vi "VT100Codes.vi"(10 "read buffer":string="\u001b[0m\u001b[01;34mmicropython-serial-0.3\u001b[0m         \u001b[01;34mrequests-2.22.0\u001b[0m\n\u001b[01;31mmicropython-serial-0.3.tar.gz\u001b[0m  \u001b[01;31mrequests-2.22.0.tar.gz\u001b[0m\nrobot@ev3dev:~$ ", 11 "Console In":string="\r\n\r\nLinux ev3dev 4.14.117-ev3dev-2.3.4-ev3 #1 PREEMPT Thu May 9 15:13:01 CDT 2019 armv5tejl\r\n             _____     _\r\n   _____   _|___ /  __| | _____   __\r\n  / _ \\ \\ / / |_ \\ / _` |/ _ \\ \\ / /\r\n |  __/\\ V / ___) | (_| |  __/\\ V /\r\n  \\___| \\_/ |____/ \\__,_|\\___| \\_/\r\n\r\nDebian stretch on LEGO MINDSTORMS EV3!\r\nLast login: Thu Feb 13 18:25:48 2020 from 130.64.189.217\r\r\nrobot@ev3dev:~$ \r\nrobot@ev3dev:~$ \r\nrobot@ev3dev:~$ brickrun -r --  pybricks-micropython\r\nPybricks MicroPython fc828f94 on 2020-01-30; linux version\r\nUse Ctrl-D to exit, Ctrl-E for paste mode\r\n>>> \nrobot@ev3dev:~$ ls\n") -> (3 "Console Out":string="\r\n\r\nLinux ev3dev 4.14.117-ev3dev-2.3.4-ev3 #1 PREEMPT Thu May 9 15:13:01 CDT 2019 armv5tejl\r\n             _____     _\r\n   _____   _|___ /  __| | _____   __\r\n  / _ \\ \\ / / |_ \\ / _` |/ _ \\ \\ / /\r\n |  __/\\ V / ___) | (_| |  __/\\ V /\r\n  \\___| \\_/ |____/ \\__,_|\\___| \\_/\r\n\r\nDebian stretch on LEGO MINDSTORMS EV3!\r\nLast login: Thu Feb 13 18:25:48 2020 from 130.64.189.217\r\r\nrobot@ev3dev:~$ \r\nrobot@ev3dev:~$ \r\nrobot@ev3dev:~$ brickrun -r --  pybricks-micropython\r\nPybricks MicroPython fc828f94 on 2020-01-30; linux version\r\nUse Ctrl-D to exit, Ctrl-E for paste mode\r\n>>> ")   [LabVIEW 2020]
uses:
  ColorText/ColorGlobals.vi
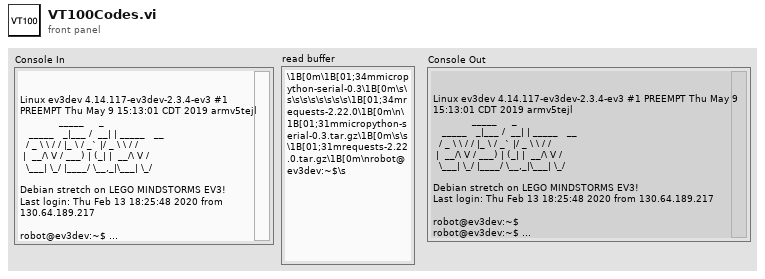
[diagram p1: front panel]
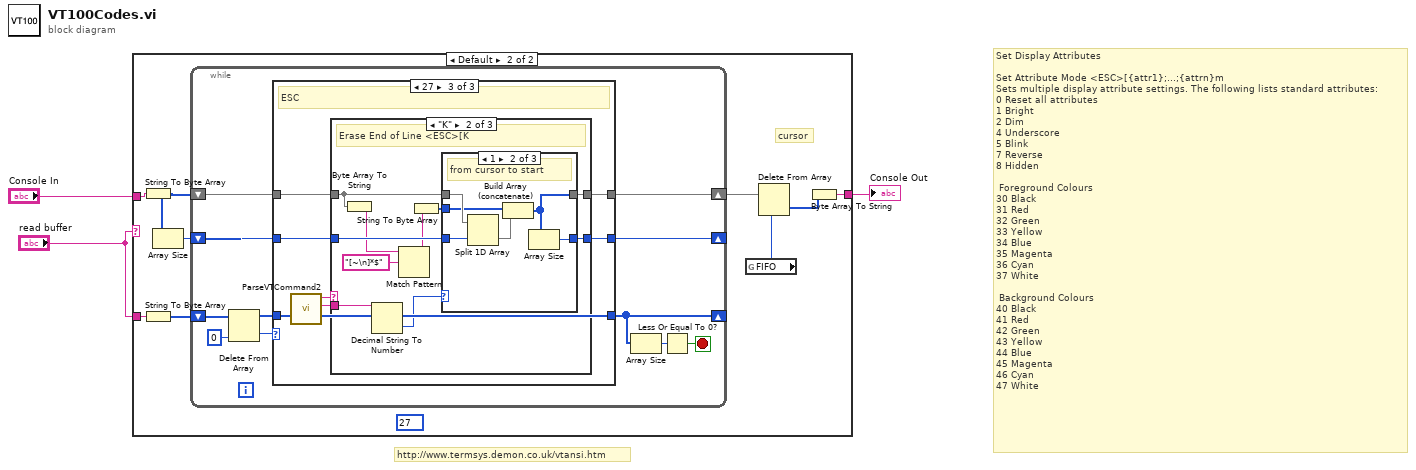
[diagram p0: block diagram]
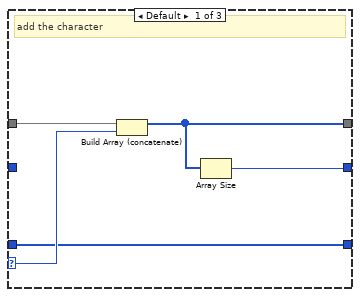
[diagram p3: hidden frame]
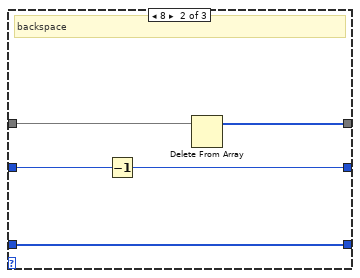
[diagram p4: hidden frame]
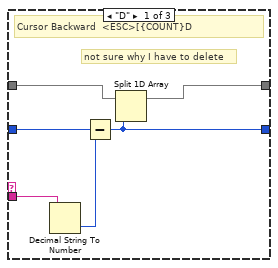
[diagram p5: hidden frame]
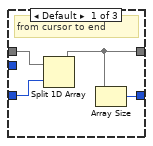
[diagram p6: hidden frame]
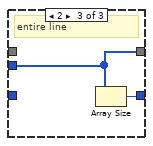
[diagram p7: hidden frame]
diagram:
  # "http://www.termsys.demon.co.uk/vtansi.htm"
  # "Set Display Attributes\n\nSet Attribute Mode\t<ESC>[{attr1};...;{attrn}m\nSets multiple display attribute settings. The following lists standard attributes:\n0\tReset all attributes\n1\tBright\n2\tDim\n4\tUnderscore\t\n5\tBlink\n7\tReverse\n8\tHidden\n\n\tForeground Colours\n30\tBlack\n31\tRed\n32\tGreen\n33\tYellow\n34\tBlue\n35\tMagenta\n36\tCyan\n37\tWhite\n\n\tBackground Colours\n40\tBlack\n41\tRed\n42\tGreen\n43\tYellow\n44\tBlue\n45\tMagenta\n46\tCyan\n47\tWhite"
  n1 = case shown="Default" "read buffer" {
    tunnel: "Console In" -> [w4 w10]
    tunnel: "read buffer" -> [_ w9]
    tunnel: [w4 w8] -> w1
    frame "" {
    }
    frame Default {
      (unwired) 27
      # "cursor"
      n2 = String To Byte Array(string=w10) -> (unsigned byte array=w12:u8[])
      n3 = String To Byte Array(string=w9) -> (unsigned byte array=w11:u8[])
      n4 = Array Size(array=w12) -> (size(s)=w13:i32)
      n5 = while {
        shift-right: [w23] -> w7
        shift-left: w12 -> [w24]
        shift-right: [w22] -> _
        shift-left: w13 -> [w21]
        shift-right: [w17] -> _
        shift-left: w11 -> [w20]
        stop <- w15 stop-if-true
        n6 = Delete From Array(array=w20, index=0) -> (deleted portion=w19:u8, array with subset deleted=w18:u8[])  [unwired: 1 in]
        n7 = case shown="27" w19 {
          selector: w19 -> [w28 _ _]
          tunnel: w24 -> [w29 w31 w39]
          tunnel: [w27 w30 w38] -> w23
          tunnel: [w26 w33 w37] -> w22
          tunnel: w21 -> [_ w34 w36]
          tunnel: [w25 w32 w41] -> w17
          tunnel: w18 -> [w25 w32 w42]
          frame Default {
            # "add the character"
            n8 = Build Array (concatenate)(w29, w28) -> (w27:u8[])
            n9 = Array Size(array=w27) -> (size(s)=w26:i32)
          }
          frame 8 {
            # "backspace"
            n10 = Decrement(x=w34) -> (x-1=w33:i32)
            n11 = Delete From Array(array=w31) -> (array with subset deleted=w30:u8[])  [unwired: 2 in, 1 out]
          }
          frame 27 {
            # "ESC"
            n12 = call "ParseVTCommand2.vi"("read buffer"=w42) -> ("VT data"=w35:string, "VT Cmd"=w40:string, "remaining"=w41:u8[])  [unwired: 6 in, 2 out]
            n13 = case shown="\"K\"" w40 {
              tunnel: w39 -> [w45 w53 w72]
              tunnel: [w43 w54 w72] -> w38
              tunnel: [w44 w56 w71] -> w37
              tunnel: w36 -> [w48 w58 w71]
              tunnel: w35 -> [w47 w57 _]
              frame "D" {
                # "not sure why I have to delete"
                # "Cursor Backward\t\t<ESC>[{COUNT}D"
                n14 = Decimal String To Number(string=w47) -> (number=w46:i32)  [unwired: 2 in, 1 out]
                n15 = Subtract(x=w48, y=w46) -> (x-y=w44:i32)
                n16 = Split 1D Array(array=w45, index=w44) -> (first subarray=w43:u8[])  [unwired: 1 out]
              }
              frame "K" {
                # "Erase End of Line\t<ESC>[K"
                n17 = Byte Array To String(unsigned byte array=w53) -> (string=w50:string)
                n18 = Decimal String To Number(string=w57) -> (number=w55:i32)  [unwired: 2 in, 1 out]
                n19 = Match Pattern(string=w50, regular expression="[~\n]*$") -> (before substring=w49:string)  [unwired: 1 in, 3 out]
                n20 = String To Byte Array(string=w49) -> (unsigned byte array=w52:u8[])
                n21 = case shown="1" w55 {
                  tunnel: w58 -> [w61 w67 _]
                  tunnel: [w60 w66 w70] -> w56
                  tunnel: [w59 w63 w69] -> w54
                  tunnel: w53 -> [w62 w68 _]
                  tunnel: w52 -> [_ w65 w69]
                  frame Default {
                    # "from cursor to end"
                    n22 = Split 1D Array(array=w62, index=w61) -> (first subarray=w59:u8[])  [unwired: 1 out]
                    n23 = Array Size(array=w59) -> (size(s)=w60:i32)
                  }
                  frame 1 {
                    # "from cursor to start"
                    n24 = Split 1D Array(array=w68, index=w67) -> (second subarray=w64:u8[])  [unwired: 1 out]
                    n25 = Build Array (concatenate)(w65, w64) -> (w63:u8[])
                    n26 = Array Size(array=w63) -> (size(s)=w66:i32)
                  }
                  frame 2 {
                    # "entire line"
                    n27 = Array Size(array=w69) -> (size(s)=w70:i32)
                  }
                }
              }
              frame Default {
              }
            }
          }
        }
        n28 = Array Size(array=w17) -> (size(s)=w16:i32)
        n29 = Less Or Equal To 0?(x=w16) -> (x <= 0?=w15:bool)
      }
      n30 = global read "ColorGlobals.vi" "FIFO"() -> (w5:i32)
      n31 = Delete From Array(array=w7, length=w5) -> (deleted portion=w6:u8[])  [unwired: 1 in, 1 out]
      n32 = Byte Array To String(unsigned byte array=w6) -> (string=w8:string)
    }
  }
  "Console Out" <- w1
